vi "From String Array.vi"(8 "error in (no error)":errorcluster, 9 "String Array":string[](array[string]), 11 "Wait Step Config in":refnum<class "Wait Step Config.lvclass">) -> (0 "error out":errorcluster, 1 "String Array 2":string[](array[string]), 2 "Version":string, 3 "Wait Step Config out":refnum<class "Wait Step Config.lvclass">)   [LabVIEW 2015, in "Wait Step Config.lvclass"]
uses:
  Wait Step Config.lvclass
  classes/Step/Config/Step Config.lvclass
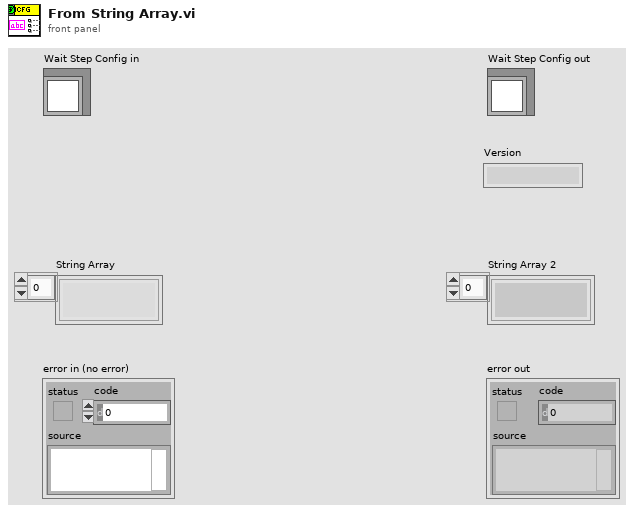
[diagram p1: front panel]
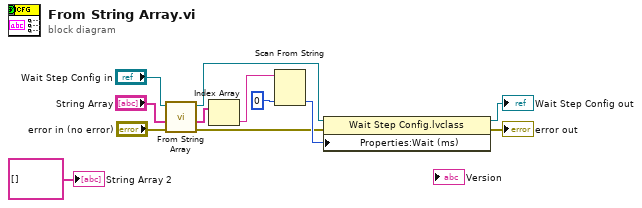
[diagram p0: block diagram]
diagram:
  n1 = call-parent "From String Array.vi"("error in (no error)"="error in (no error)", "String Array"="String Array", "Step Config in"="Wait Step Config in") -> ("error out"=w6:errorcluster, "Elements Left"=w3:string[], "Step Config out"=w5:refnum<class "Wait Step Config.lvclass">)  [unwired: 5 in, 1 out]
  n2 = Index Array(array=w3) -> (element=w1:string)  [unwired: 1 in]
  n3 = Scan From String(input string=w1, default 1=u32 0 ("Wait (ms)")) -> (output 1=w9:u32)  [unwired: 3 in, 3 out]
  n4 = property class="Wait Step Config.lvclass"(reference=w5, error in=w6, "Properties:Wait (ms)"=w9) -> (reference out=→"Wait Step Config out":refnum<class "Wait Step Config.lvclass">, error out=→"error out":errorcluster)
  "String Array 2" <- string[] [] ("String Array 2")
